vi "Initialize Attributes.vi"(8 "error in (no error)":errorcluster, 10 "Attribute Data":variant, 11 "CS++Base in":refnum<class "CS++Base.lvclass">) -> (0 "error out":errorcluster, 2 "Found?":bool, 3 "CS++Base out":refnum<class "CS++Base.lvclass">)   [LabVIEW 2016, in "CS++BaseClasses.lvlib" / "CS++Base.lvclass"]
doc: "Initialize object attribute.\n\nUnique resources should be allocated elsewhere!"
uses:
  CS++Base.lvclass
  CS++Base.lvclass/CS++Base.ctl
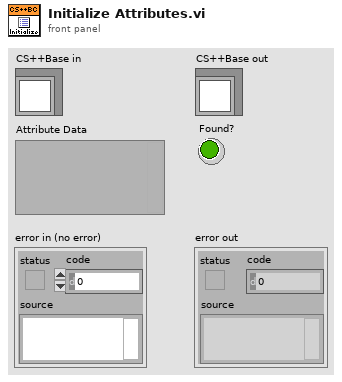
[diagram p1: front panel]
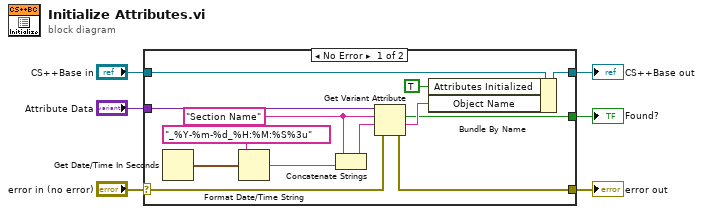
[diagram p0: block diagram]
diagram:
  n1 = case shown="No Error" "error in (no error)" {
    selector: "error in (no error)" -> [w13 w21]
    tunnel: [w12 w21] -> w5
    tunnel: [w18 w20] -> w3
    tunnel: "CS++Base in" -> [w19 w20]
    tunnel: "Attribute Data" -> [w17 _]
    tunnel: [w8 _] -> w1
    frame No Error {
      w10 = "Section Name" ("name")
      n2 = Get Date/Time In Seconds() -> (seconds since 1Jan1904=w16:timestamp)
      n3 = Format Date/Time String(time format string (%c)="_%Y-%m-%d_%H:%M:%S%3u", seconds (now)=w16) -> (date/time string=w14:string)  [unwired: 1 in]
      n4 = Concatenate Strings(w10, w14) -> (w11:string)
      n5 = Get Variant Attribute(Variant=w17, name=w10, default value (empty Variant)=w11, error in=w13) -> (found=w8:bool, value=w9:string, error out=w12:errorcluster)  [unwired: 1 out]
      n6 = Bundle By Name(cluster=w19, "Attributes Initialized"=TRUE, "Object Name"=w9) -> (w18:refnum<class "CS++Base.lvclass">)
    }
    frame Error {
    }
  }
  "error out" <- w5
  "CS++Base out" <- w3
  "Found?" <- w1
